vi "green.vi"(0 "Image In":T2, 1 "ROI Descriptor (Line Profile 1)":T1={"Global Rectangle"=[100, 292, 131, 371], "Contours"=[{"ID"=enum."External", "Type"=2, "Coordinates"=[100, 370, 130, 292]}]} {"Contours"."Type" items=["No Selection", "Point", "Line", "Rectangle", "Oval", "Polygon", "Freehand Region", "Annulus", "Unused2", "Unused3", "Broken Line", "Freehand Line", "Rotated Rectangle"]}, 7 "error in":errorcluster) -> (20 "Image Out":T2, 27 "error out":errorcluster)   [LabVIEW 2009]
uses:
  <vilib>/vision/Image Controls.llb/IMAQ Image.ctl
panel:
  out "Line Profile Graph":u8[][](graph) caption="Line Profile"
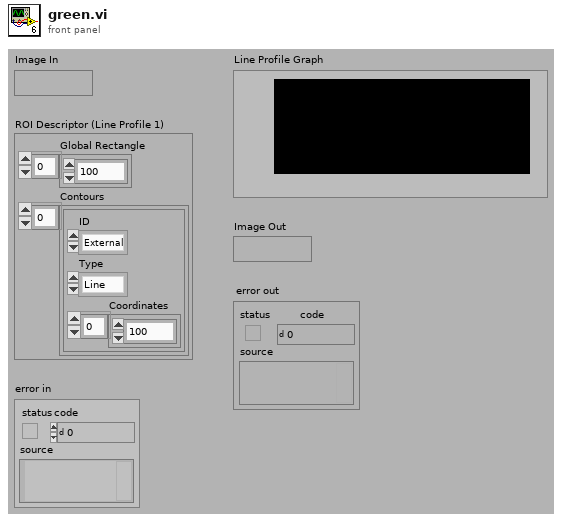
[diagram p1: front panel]
types:
  T1 = cluster{"Global Rectangle":i32[], "Contours":cluster{"ID":enum32{"External", "Internal"}, "Type":u32, "Coordinates":i32[]}[]}
  T2 = typedef "IMAQ Image.ctl" = refnum<image>
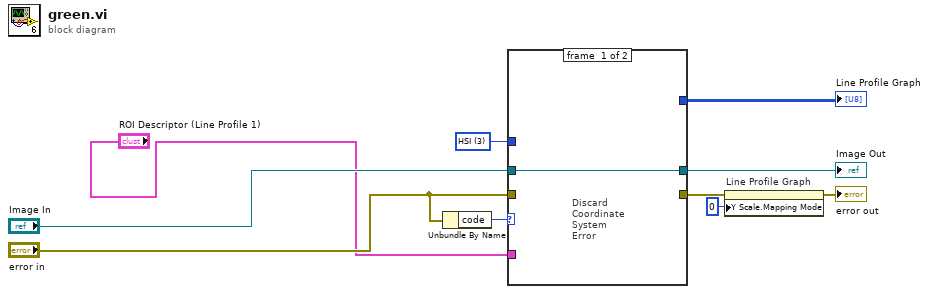
[diagram p0: block diagram]
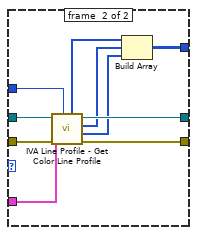
[diagram p2: hidden frame]
diagram:
  w6 = u16 3 items=["RGB", "HSL", "HSV", "HSI"] ("Color Mode")
  n1 = Unbundle By Name("error in") -> ("code"=w1:i32)
  n2 = case shown="Default" w1 {
    tunnel: "error in" -> [_ w21]
    tunnel: [_ w20] -> w8
    tunnel: w6 -> [_ w19]
    tunnel: [w11 w18] -> w5
    tunnel: "Image In" -> [w11 w17]
    tunnel: [_ w13] -> w3
    tunnel: "ROI Descriptor (Line Profile 1)" -> [_ w12]
    frame #0 {
      # "Discard\nCoordinate\nSystem\nError"
    }
    frame #1 {
      n3 = call <vilib>:"IVA Line Profile - Get Color Line Profile.vi"("Color Mode"=w19, "error in (no error)"=w21, "ROI Descriptor"=w12, "Image In"=w17) -> ("error out"=w20:errorcluster, "Blue or Luma Pixels"=w14:u8[], "Green or Sat Pixels"=w15:u8[], "Image Out"=w18:T2, "Red or Hue Pixels"=w16:u8[])  [unwired: 3 out]
      n4 = Build Array(w16, w15, w14) -> (w13:u8[][])
    }
  }
  "Line Profile Graph" <- w3
  "Image Out" <- w5
  n5 = property on="Line Profile Graph"(error in=w8, "Y Scale.Mapping Mode"=u8 0) -> (error out=→"error out":errorcluster)  [unwired: 1 in, 1 out]
